vi "GEOM_SetNampsxy.vi"(10 "BinFPA":T1, 11 "Database RefNum in":T2) -> ()   [LabVIEW 2016]
uses:
  DBSHAND/private/vis/DatabaseHand_RefNum.ctl
  GEOM_CorrectedFPA.ctl
  DBSHAND/private/vis/DatabaseHand_Element_Set(string).vi
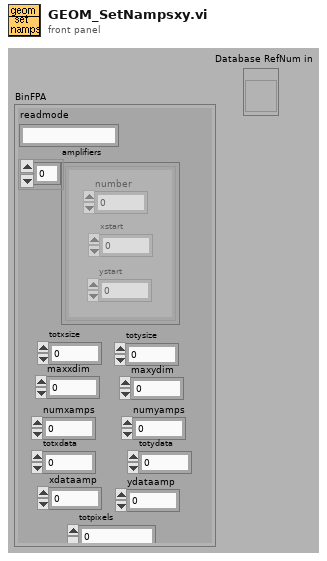
[diagram p1: front panel]
types:
  T1 = typedef "GEOM_CorrectedFPA.ctl" = cluster{"readmode":string, "amplifiers":cluster{"number":i32, "xstart":i32, "ystart":i32}[], "totxsize":i32, "totysize":i32, "maxxdim":i32, "maxydim":i32, "numxamps":i32, "numyamps":i32, "totxdata":i32, "totydata":i32, "xdataamp":i32, "ydataamp":i32, "totpixels":i32}
  T2 = typedef "DatabaseHand_RefNum.ctl" = refnum<vi>
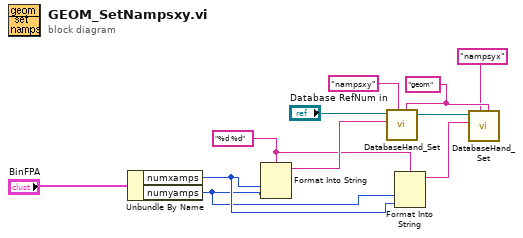
[diagram p0: block diagram]
diagram:
  w5 = "%d %d" ("format string")
  w7 = "geom" ("group")
  n1 = Unbundle By Name("BinFPA") -> ("numxamps"=w4:i32, "numyamps"=w3:i32)
  n2 = Format Into String(format string=w5, w4, w3) -> (resulting string=w9:string)  [unwired: 2 in, 1 out]
  n3 = call-poly "DatabaseHand_Set.vi"("group"=w7, "name"="nampsxy", "value"=w9, "Database RefNum in"="Database RefNum in") -> ("Database RefNum out"=w1:T2)  [unwired: 4 in, 3 out]
  n4 = Format Into String(format string=w5, w3, w4) -> (resulting string=w2:string)  [unwired: 2 in, 1 out]
  n5 = call-poly "DatabaseHand_Set.vi"("group"=w7, "name"="nampsyx", "value"=w2, "Database RefNum in"=w1) -> ()  [unwired: 4 in, 4 out]
